vi "CalculateMatrixPoint.vi"(0 "object in":refnum<class "Evaluator.lvclass">, 2 "GameRef":refnum<data-value>, 5 "error in (no error)":errorcluster) -> (14 "object out":refnum<class "Evaluator.lvclass">, 16 "output array":dbl[][](array[numeric]), 19 "error out":errorcluster)   [LabVIEW 2023, in "Evaluator.lvclass"]
uses:
  Evaluator.lvclass
  Game_class/Game.lvclass
  Evaluator.lvclass/Evaluator.ctl
  Game_class/Game.lvclass/Game.ctl
  Game_class/Read FieldRef.vi
  Field_class/Field.lvclass
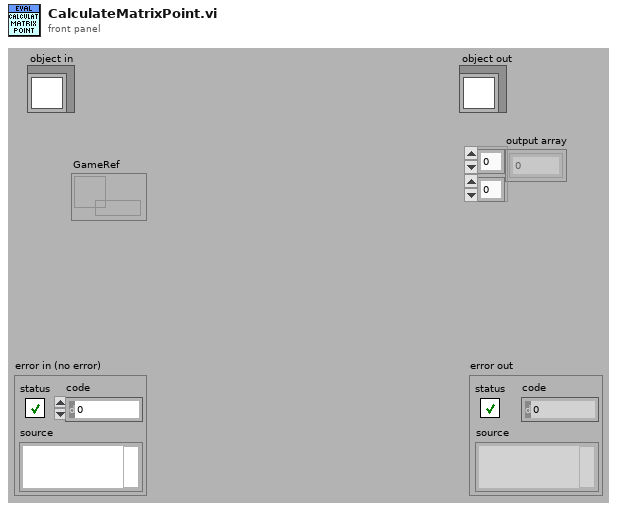
[diagram p1: front panel]
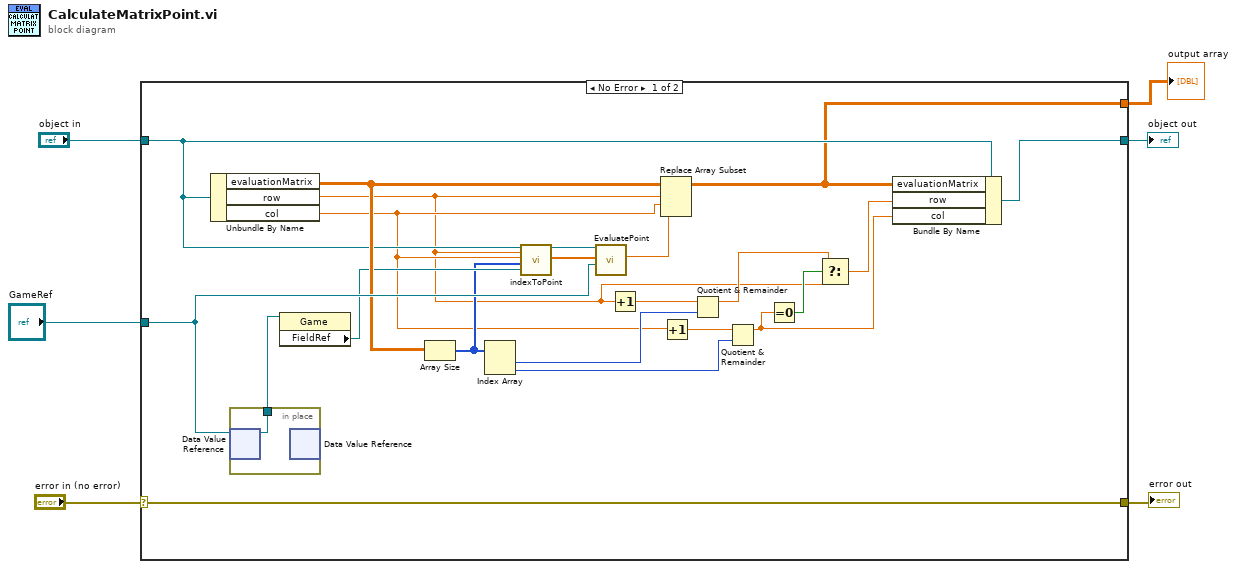
[diagram p0: block diagram]
diagram:
  n1 = case shown="No Error" "error in (no error)" {
    selector: "error in (no error)" -> [w28 w31]
    tunnel: [w28 w31] -> w5
    tunnel: [w20 w30] -> w3
    tunnel: "object in" -> [w19 w30]
    tunnel: "GameRef" -> [w27 _]
    tunnel: [w15 _] -> w2
    frame No Error {
      n2 = Unbundle By Name(w19) -> ("evaluationMatrix"=w24:dbl[][], "row"=w9:dbl, "col"=w13:dbl)
      n3 = in-place {
        in-place-border: [w29] -> w26
        n4 = in-place-dvr #1(w27) -> (w29:refnum<class "Game.lvclass">)  [unwired: 1 out]
        n5 = in-place-dvr #1() -> ()  [unwired: 1 in, 2 out]
      }
      n6 = property class="Game"(reference=w26) -> ("FieldRef"=w17:refnum<class "Field.lvclass">)  [unwired: 1 in, 2 out]
      n7 = Array Size(array=w24) -> (size(s)=w14:i32[])
      n8 = Index Array(array=w14) -> (element #1=w22:i32, element #2=w21:i32)  [unwired: 2 in]
      n9 = call "indexToPoint.vi"("object in"=w19, "row"=w9, "col"=w13, "matrixSize"=w14, "Field"=w17) -> ("object out"=w18:refnum<class "Evaluator.lvclass">, "point"=w16:dbl[])  [unwired: 12 in, 1 out]
      n10 = call-dynamic "EvaluatePoint.vi"("GameRef"=w27, "Point"=w16, "Evaluator in"=w18) -> ("Evaluation"=w7:dbl)  [unwired: 6 in, 2 out]
      n11 = Increment(x=w9) -> (x+1=w23:dbl)
      n12 = Replace Array Subset(array=w24, new element=w7, index (row)=w9, index (col)=w13) -> (w15:dbl[][])
      n13 = Increment(x=w13) -> (x+1=w25:dbl)
      n14 = Quotient & Remainder(x=w23, y=w22) -> (x-y*floor(x/y)=w10:dbl)  [unwired: 1 out]
      n15 = Quotient & Remainder(x=w25, y=w21) -> (x-y*floor(x/y)=w11:dbl)  [unwired: 1 out]
      n16 = Equal To 0?(x=w11) -> (x = 0?=w12:bool)
      n17 = Select(t=w10, s=w12, f=w9) -> (s? t:f=w8:dbl)
      n18 = Bundle By Name(cluster=w19, "evaluationMatrix"=w15, "row"=w8, "col"=w11) -> (w20:refnum<class "Evaluator.lvclass">)
    }
    frame Error {
    }
  }
  "error out" <- w5
  "object out" <- w3
  "output array" <- w2
